vi "ESP301_PA.vi"(8 "position":dbl, 10 "axisNumber":i32=1, 11 "COM_PORT":string="COM12") -> (0 "errstring":string)   [LabVIEW 2019]
uses:
  Newport.ESP301.CommandInterface
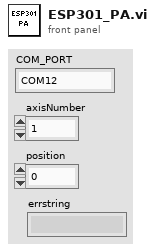
[diagram p1: front panel]
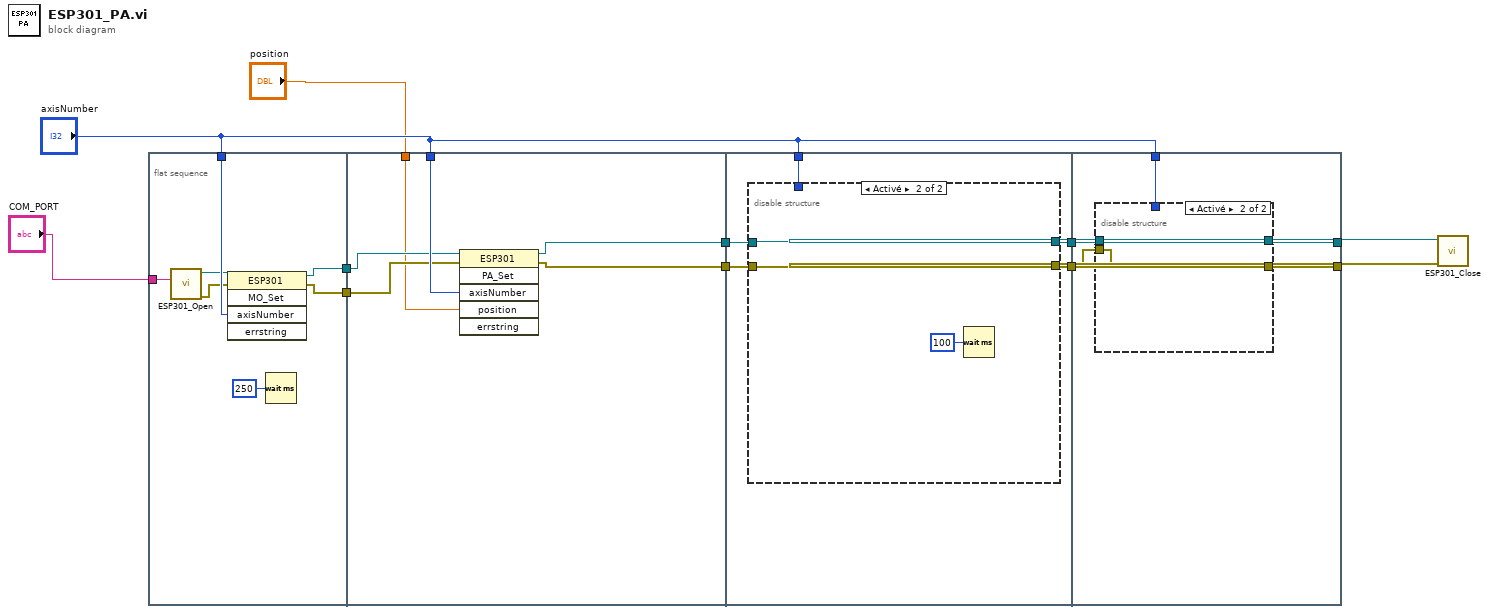
[diagram p0: block diagram]
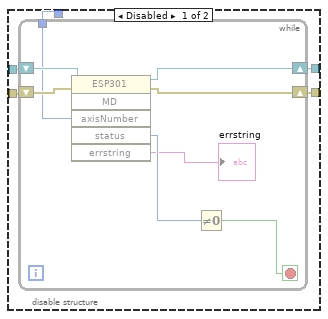
[diagram p2: hidden frame]
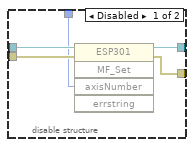
[diagram p3: hidden frame]
diagram:
  n1 = flat-sequence {
    tunnel: [w13] -> w9
    tunnel: [w14] -> w8
    tunnel: "COM_PORT" -> [w18]
    tunnel: "axisNumber" -> [w17]
    tunnel: "axisNumber" -> [w24]
    tunnel: w9 -> [w21]
    tunnel: w8 -> [w20]
    tunnel: [w23] -> w6
    tunnel: [w22] -> w5
    tunnel: "position" -> [w19]
    tunnel: w6 -> [w28]
    tunnel: w5 -> [w27]
    tunnel: [w26] -> w4
    tunnel: [w25] -> w3
    tunnel: "axisNumber" -> [w29]
    tunnel: [w47] -> w10
    tunnel: [w48] -> w11
    tunnel: w4 -> [w50]
    tunnel: w3 -> [w49]
    tunnel: "axisNumber" -> [w46]
    frame #0 {
      n2 = call "ESP301_Open.vi"("strDeviceKey"=w18) -> ("sortie d'erreur"=w15:errorcluster, "référence en sortie"=w16:refnum<k24>)  [unwired: 9 in]
      n3 = invoke on="Nœud de méthode" class="ESP301" method="MO_Set"(reference=w16, error in=w15, "axisNumber"=w17) -> (reference out=w14:refnum<k24>, error out=w13:errorcluster)  [unwired: 2 in, 3 out]
      n4 = Wait (ms)(milliseconds to wait=u32 250 ("attente (ms)")) -> ()  [unwired: 1 out]
    }
    frame #1 {
      n5 = invoke on="Nœud de méthode" class="ESP301" method="PA_Set"(reference=w20, error in=w21, "axisNumber"=w24, "position"=w19) -> (reference out=w23:refnum<k24>, error out=w22:errorcluster)  [unwired: 2 in, 4 out]
    }
    frame #2 {
      n6 = disable-structure shown="Activé" {
        disable-tunnel: w29 -> [w34 _]
        disable-tunnel: w28 -> [w33 w45]
        disable-tunnel: w27 -> [w32 w44]
        disable-tunnel: [w31 w45] -> w26
        disable-tunnel: [w30 w44] -> w25
        frame Disabled {
          n7 = while {
            tunnel: w34 -> [w40]
            shift-right: [w39] -> w31
            shift-left: w33 -> [w42]
            shift-right: [w38] -> w30
            shift-left: w32 -> [w41]
            stop <- w37 stop-if-true
            n8 = invoke on="Nœud de méthode" class="ESP301" method="MD"(reference=w42, error in=w41, "axisNumber"=w40) -> (reference out=w39:refnum<k24>, error out=w38:errorcluster, "status"=w36:i32, "errstring"=→"errstring":string)  [unwired: 3 in, 2 out]
            n9 = Not Equal To 0?(x=w36) -> (x != 0?=w37:bool)
          }
        }
        frame Enabled {
          n10 = Wait (ms)(milliseconds to wait=u32 100 ("attente (ms)")) -> ()  [unwired: 1 out]
        }
      }
    }
    frame #3 {
      n11 = disable-structure shown="Activé" {
        disable-tunnel: w50 -> [w55 w57]
        disable-tunnel: w49 -> [w54 w56]
        disable-tunnel: [w53 w57] -> w48
        disable-tunnel: [w52 w56] -> w47
        disable-tunnel: w46 -> [w51 _]
        frame Disabled {
          n12 = invoke on="Nœud de méthode" class="ESP301" method="MF_Set"(reference=w55, error in=w54, "axisNumber"=w51) -> (reference out=w53:refnum<k24>, error out=w52:errorcluster)  [unwired: 2 in, 3 out]
        }
        frame Enabled {
        }
      }
    }
  }
  n13 = call "ESP301_Close.vi"("entrée d'erreur (pas d'erreur)"=w10, "référence"=w11) -> ()  [unwired: 9 in, 1 out]
